vi "Rotation3d_Create_Default.vi"() -> (3 "ROTATION3D":T1={"Q_quaternion"={"R"=1.0, "V"=[0.0, 0.0, 0.0]}})   [LabVIEW 2019, in "Trajectory_Library.lvlib"]
doc: "Constructs a Rotation2d with the given radian value. The x and y don't have to be normalized.\n\nParmeters:\n - value - The value of the angle in radians.\n\nReturns\n - rotation data structure"
uses:
  Trajectory_Library.lvlib
  ROTATION3D.ctl
  QUATERNION.ctl
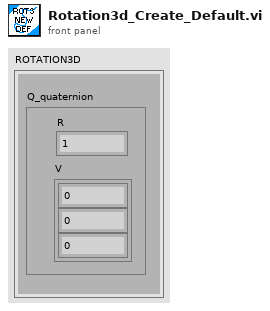
[diagram p1: front panel]
types:
  T1 = typedef "Trajectory_Library.lvlib/ROTATION3D.ctl" = cluster{"Q_quaternion":T2}
  T2 = typedef "Trajectory_Library.lvlib/QUATERNION.ctl" = cluster{"R":dbl, "V":dbl[]}
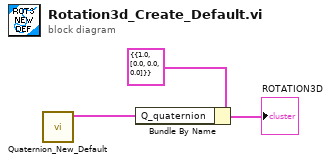
[diagram p0: block diagram]
diagram:
  n1 = call "Quaternion_New_Default.vi"() -> ("out Quaternion"=w1:T2)  [unwired: 11 in]
  n2 = Bundle By Name(cluster=T1 {"Q_quaternion"={"R"=1.0, "V"=[0.0, 0.0, 0.0]}} ("ROTATION3D"), "Q_quaternion"=w1) -> (→"ROTATION3D":T1)
